vi "CountShantenWithEye.vi"(1 "HandCount":u16[](array[numeric])) -> (0 "Max":u16)   [LabVIEW 2025]
panel:
  in  "HandCount 2":u16[](array[numeric])
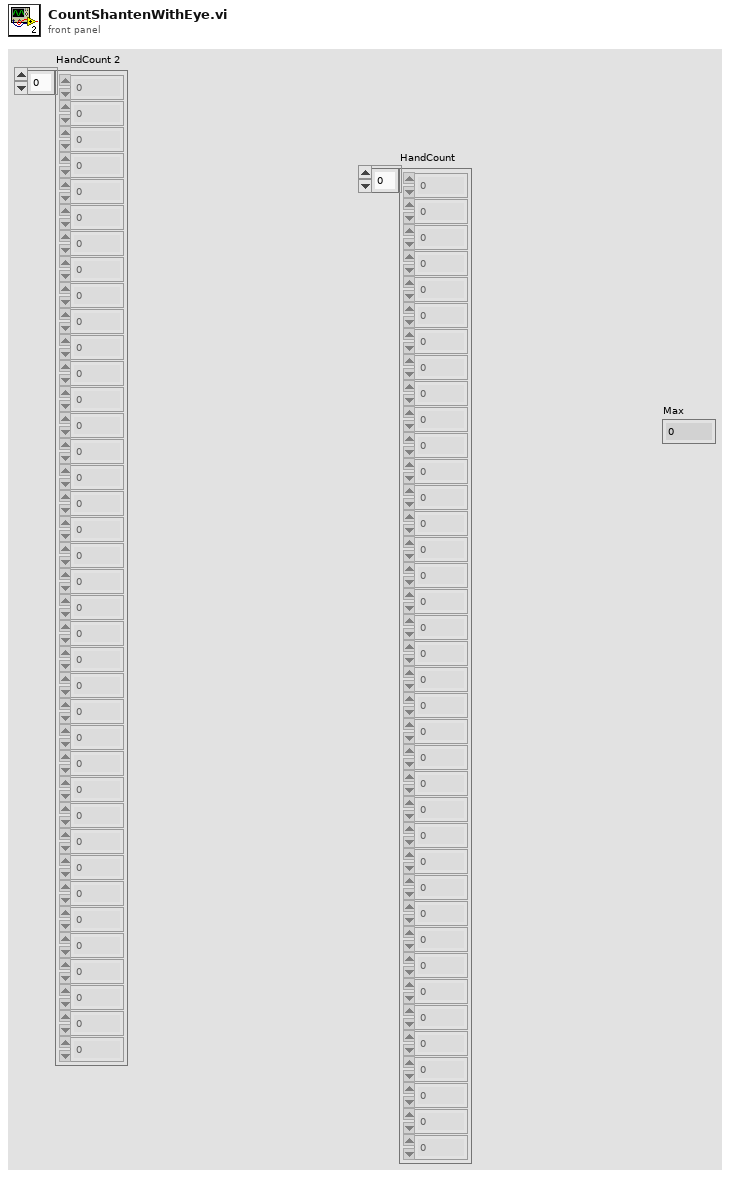
[diagram p1: front panel]
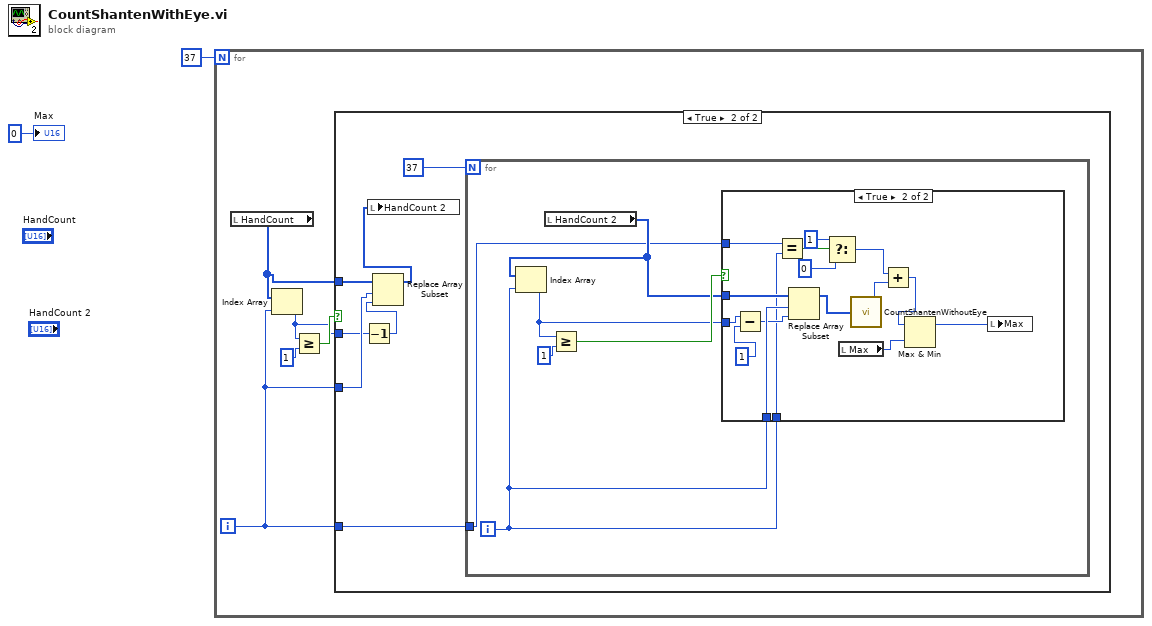
[diagram p0: block diagram]
diagram:
  n1 = for {
    N: 37 -> [_]
    i -> [w3]
    n2 = local read "HandCount"() -> (w5:u16[])
    n3 = Index Array(array=w5, index=w3) -> (element=w4:u16)
    n4 = Greater Or Equal?(x=w4, y=1) -> (x >= y?=w6:bool)
    n5 = case shown="True" w6 {
      tunnel: w5 -> [_ w13]
      tunnel: w3 -> [_ w12]
      tunnel: w4 -> [_ w10]
      tunnel: w3 -> [_ w8]
      frame False {
      }
      frame True {
        n6 = Decrement(x=w10) -> (x-1=w11:u16)
        n7 = Replace Array Subset(array=w13, new element=w11, index=w12) -> (w9:u16[])
        n8 = local write "HandCount 2"(w9) -> ()
        n9 = for {
          N: 37 -> [_]
          tunnel: w8 -> [w15]
          i -> [w16]
          n10 = local read "HandCount 2"() -> (w17:u16[])
          n11 = Index Array(array=w17, index=w16) -> (element=w18:u16)
          n12 = Greater Or Equal?(x=w18, y=1) -> (x >= y?=w20:bool)
          n13 = case shown="True" w20 {
            tunnel: w16 -> [_ w36]
            tunnel: w17 -> [_ w35]
            tunnel: w18 -> [_ w33]
            tunnel: w16 -> [_ w27]
            tunnel: w15 -> [_ w26]
            frame False {
            }
            frame True {
              n14 = Subtract(x=w33, y=1) -> (x-y=w34:i32)
              n15 = Equal?(x=w26, y=w27) -> (x = y?=w28:bool)
              n16 = Replace Array Subset(array=w35, new element=w34, index=w36) -> (w31:u16[])
              n17 = Select(t=u16 1, s=w28, f=u16 0) -> (s? t:f=w23:u16)
              n18 = local read "Max"() -> (w30:u16)
              n19 = call "CountShantenWithoutEye.vi"("HandCount"=w31) -> ("shanten"=w22:u16)
              n20 = Add(x=w23, y=w22) -> (x+y=w21:u16)
              n21 = Max & Min(x=w21, y=w30) -> (max(x,y)=w29:u16)  [unwired: 1 out]
              n22 = local write "Max"(w29) -> ()
            }
          }
        }
      }
    }
  }
  "Max" <- u16 0 ("Numeric")
